vi "Slack-Write Config.vi"(0 "AppName":path, 5 "config":T2, 7 "users":T1[](array[typedef]), 11 "Error In":errorcluster) -> (15 "error out":errorcluster)   [LabVIEW 2020]
uses:
  Typedefs/Slack-Configuration.ctl
  Typedefs/Slack-User.ctl
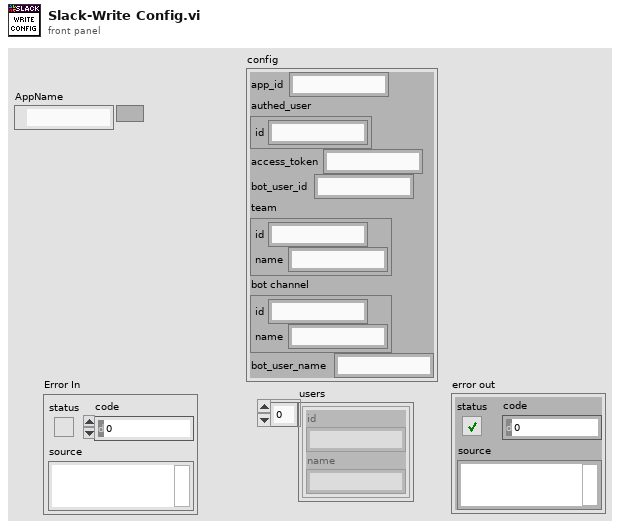
[diagram p1: front panel]
types:
  T1 = typedef "Slack-User.ctl" = cluster{"id":string, "name":string}
  T2 = typedef "Slack-Configuration.ctl" = cluster{"app_id":string, "authed_user":cluster{"id":string}, "access_token":string, "bot_user_id":string, "team":cluster{"id":string, "name":string}, "bot channel":cluster{"id":string, "name":string}, "bot_user_name":string}
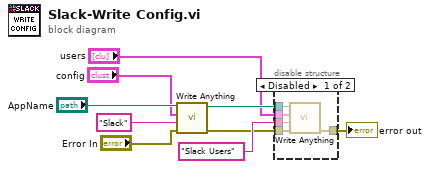
[diagram p0: block diagram]
diagram:
  n1 = call "Write Anything.vi"("Error In"="Error In", "Section Name (Name of \"Anything\")"="Slack" ("Section Name (Name of \"Type of Anything\")"), "Anything"="config", "Path (dialog)"="AppName") -> ("Error Out"=w4:errorcluster, "Path out"=w3:path)  [unwired: 6 in]
  n2 = disable-structure shown="Disabled" {
    disable-tunnel: "Slack Users" ("Section Name (Name of \"Type of Anything\")") -> [w14 _]
    disable-tunnel: w4 -> [w13 w15]
    disable-tunnel: w3 -> [w12 _]
    disable-tunnel: "users" -> [w11 _]
    disable-tunnel: [w10 w15] -> w1
    frame Disabled {
      n3 = call "Write Anything.vi"("Error In"=w13, "Section Name (Name of \"Anything\")"=w14, "Anything"=w11, "Path (dialog)"=w12) -> ("Error Out"=w10:errorcluster)  [unwired: 6 in, 1 out]
    }
    frame Enabled {
    }
  }
  "error out" <- w1
